vi "svfa_Spectrum to Spectral Density.vi"(0 "input signal":dbl[](array[numeric]) format="%.2f", 1 "spectral density desired":T1(ring), 2 "df":dbl format="%.2f", 3 "window size":i32, 5 "linear/dB":enum16{"linear", "dB"}(ring), 7 "power/magnitude":enum16{"power", "magnitude"}(ring), 9 "view":enum16{"rms", "peak", "peak-peak"}(ring), 11 "dB reference":dbl format="%.2f", 12 "spectral density?":bool, 13 "window":u16(ring) items=["None ", "Hanning", "Hamming", "Blackman-Harris", "Exact Blackman", "Blackman", "Flat Top", "4 Term B-Harris ", "7 Term B-Harris", "Low Sidelobe"]) -> (4 "converted signal":dbl[](array[numeric]) format="%.2f", 6 "dup linear/dB":enum16{"linear", "dB"}(ring), 8 "power/magnitude (dupl)":enum16{"power", "magnitude"}(ring), 10 "dup view":enum16{"rms", "peak", "peak-peak"}(ring), 14 "spectral density?":bool, 15 "dB reference (out)":dbl format="%.2f")   [LabVIEW 2017]
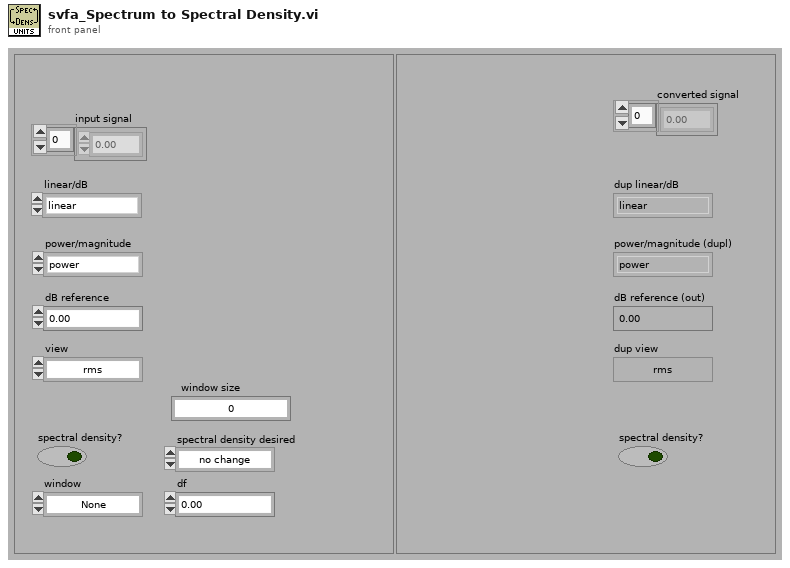
[diagram p1: front panel]
types:
  T1 = enum16{"no change", "spectrum", "spectral density"}
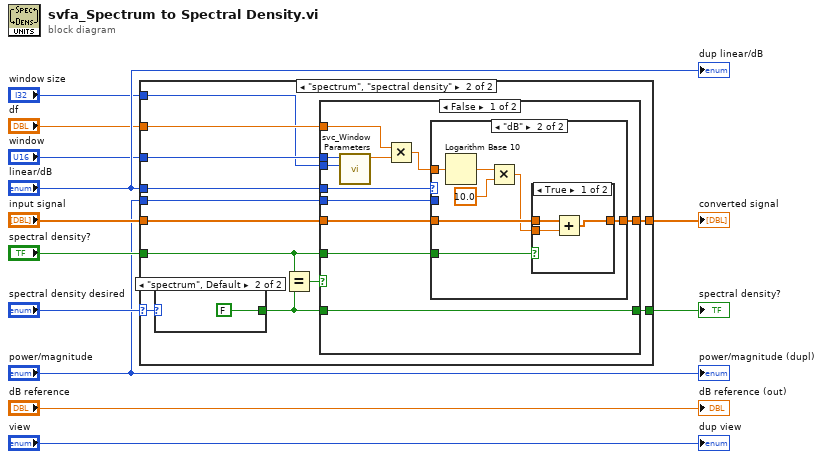
[diagram p0: block diagram]
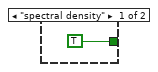
[diagram p3: hidden frame]
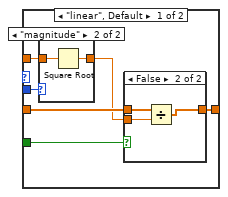
[diagram p4: hidden frame]
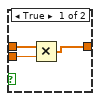
[diagram p5: hidden frame]
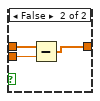
[diagram p7: hidden frame]
diagram:
  n1 = case shown="\"spectrum\", \"spectral density\"" "spectral density desired" {
    selector: "spectral density desired" -> [_ w21]
    tunnel: [w13 w26] -> w12
    tunnel: [w14 w25] -> w11
    tunnel: "linear/dB" -> [_ w24]
    tunnel: "spectral density?" -> [w13 w20]
    tunnel: "input signal" -> [w14 w23]
    tunnel: "window" -> [_ w19]
    tunnel: "df" -> [_ w18]
    tunnel: "power/magnitude" -> [_ w17]
    tunnel: "window size" -> [_ w15]
    frame "no change", Default {
    }
    frame "spectrum", "spectral density" {
      n2 = case shown="\"spectrum\", Default" w21 {
        tunnel: [TRUE FALSE] -> w16
        frame "spectral density" {
        }
        frame "spectrum", Default {
        }
      }
      n3 = Equal?(x=w20, y=w16) -> (x = y?=w22:bool)
      n4 = case shown="False" w22 {
        tunnel: w23 -> [w38 w69]
        tunnel: [w37 w69] -> w25
        tunnel: w24 -> [w39 _]
        tunnel: [w36 w68] -> w26
        tunnel: w16 -> [w36 w68]
        tunnel: w20 -> [w35 _]
        tunnel: w19 -> [w33 _]
        tunnel: w18 -> [w32 _]
        tunnel: w17 -> [w30 _]
        tunnel: w15 -> [w29 _]
        frame False {
          n5 = call <vilib>:"svc_Window Parameters.vi"("window size"=w29, "window"=w33) -> ("ENBW"=w34:dbl)  [unwired: 6 in, 3 out]
          n6 = Multiply(x=w32, y=w34) -> (x*y=w31:dbl)
          n7 = case shown="\"dB\"" w39 {
            tunnel: w38 -> [w43 w61]
            tunnel: [w41 w60] -> w37
            tunnel: w35 -> [w40 w55]
            tunnel: w31 -> [w45 w59]
            tunnel: w30 -> [w44 _]
            frame "linear", Default {
              n8 = case shown="\"magnitude\"" w44 {
                tunnel: w45 -> [w52 w53]
                tunnel: [w52 w54] -> w42
                frame "power", Default {
                }
                frame "magnitude" {
                  n9 = Square Root(x=w53) -> (sqrt(x)=w54:dbl)
                }
              }
              n10 = case shown="False" w40 {
                tunnel: w43 -> [w48 w51]
                tunnel: [w47 w50] -> w41
                tunnel: w42 -> [w46 w49]
                frame True {
                  n11 = Multiply(x=w48, y=w46) -> (x*y=w47:dbl[])
                }
                frame False {
                  n12 = Divide(x=w51, y=w49) -> (x/y=w50:dbl[])
                }
              }
            }
            frame "dB" {
              n13 = Logarithm Base 10(1:w59) -> (0:w58:dbl)
              n14 = Multiply(x=w58, y=10.0) -> (x*y=w56:dbl)
              n15 = case shown="True" w55 {
                tunnel: w61 -> [w64 w67]
                tunnel: [w63 w66] -> w60
                tunnel: w56 -> [w62 w65]
                frame True {
                  n16 = Add(x=w64, y=w62) -> (x+y=w63:dbl[])
                }
                frame False {
                  n17 = Subtract(x=w67, y=w65) -> (x-y=w66:dbl[])
                }
              }
            }
          }
        }
        frame True {
        }
      }
    }
  }
  "spectral density?" <- w12
  "converted signal" <- w11
  "dup linear/dB" <- "linear/dB"
  "dup view" <- "view"
  "dB reference (out)" <- "dB reference"
  "power/magnitude (dupl)" <- "power/magnitude"
